vi "Get Sub-Item Type Descriptor.vi"(9 "error in (no error)":errorcluster, 10 ".NET AdsDataType":refnum<k24>) -> (1 "error out":errorcluster, 2 ".NET AdsDataType":refnum<k24>, 3 "[Sub-Item Type Descriptor]":T1[](array[typedef]))   [LabVIEW 2018, in "TwinCAT ADS.lvclass"]
uses:
  TwinCAT ADS.lvclass
  TwinCAT.Ads
  Controls/PLC Sub-Item Type Descriptor.ctl
  Controls/PLC Type.ctl
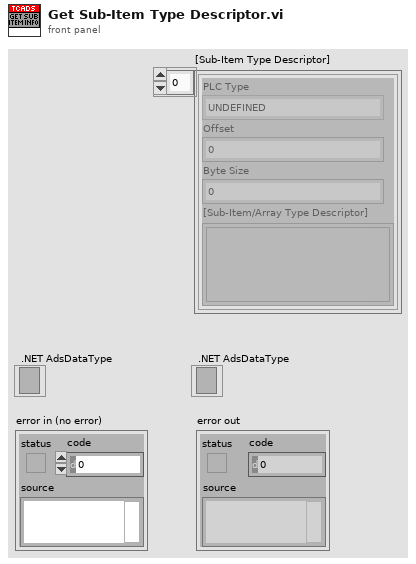
[diagram p1: front panel]
types:
  T1 = typedef "TwinCAT ADS.lvclass/PLC Sub-Item Type Descriptor.ctl" = cluster{"PLC Type":T2, "Offset":i32, "Byte Size":i32, "[Sub-Item/Array Type Descriptor]":variant[]}
  T2 = typedef "TwinCAT ADS.lvclass/PLC Type.ctl" = enum16{"UNDEFINED", "INT", "DINT", "REAL", "LREAL", "SINT", "BYTE", "UINT", "UDINT", "LINT", "ULINT", "STRING", "WSTRING", "BOOL", "TIME", "LTIME", "DATE", "DT", "TOD", "ARRAY", "JAGGED ARRAY", "STRUCT", "FUNCTION BLOCK", "POINTER", "USER DEFINED"}
  T3 = typedef "TwinCAT ADS.lvclass/PLC Array Type Descriptor.ctl" = cluster{"Fundamental PLC Type":T2, "Fundamental Type Byte Size":i32, "Item Count":i32, "Dimension Lengths":i32[], "Sub-Item Type Descriptor":variant}
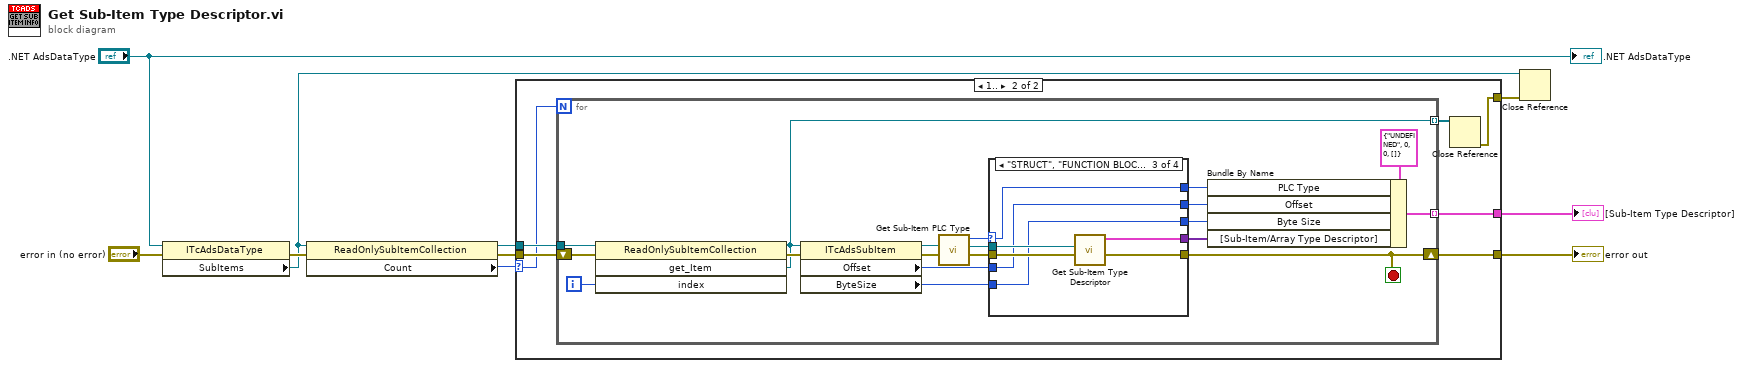
[diagram p0: block diagram]
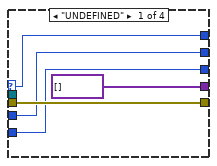
[diagram p3: hidden frame]
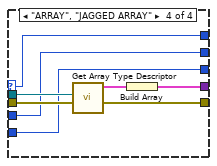
[diagram p5: hidden frame]
diagram:
  n1 = property class="ITcAdsDataType"(reference=".NET AdsDataType", error in="error in (no error)") -> (error out=w10:errorcluster, "SubItems"=w1:refnum<k24>)  [unwired: 1 out]
  n2 = property class="ReadOnlySubItemCollection"(reference=w1, error in=w10) -> (reference out=w7:refnum<k24>, error out=w8:errorcluster, "Count"=w4:i32)
  n3 = case shown="1.." w4 {
    selector: w4 -> [_ w14]
    tunnel: w8 -> [w11 w18]
    tunnel: w7 -> [_ w17]
    tunnel: [w11 w16] -> w6
    tunnel: [_ w15] -> w5
    tunnel: [_ w12] -> w2
    frame Default {
    }
    frame 1.. {
      n4 = for {
        N: w14 -> [_]
        shift-right: [w20] -> w16
        shift-left: w18 -> [w37]
        tunnel: w17 -> [w35]
        tunnel: [w26] -> w15 mode=indexing
        tunnel: [w21] -> w13 mode=indexing
        i -> [w36]
        stop <- w20 stop-if-true
        n5 = invoke class="ReadOnlySubItemCollection" method="get_Item"(reference=w35, error in=w37, "index"=w36) -> (error out=w34:errorcluster, "get_Item"=w21:refnum<k24>)  [unwired: 1 in, 2 out]
        n6 = property class="ITcAdsSubItem"(reference=w21, error in=w34) -> (reference out=w32:refnum<k24>, error out=w33:errorcluster, "Offset"=w19:i32, "ByteSize"=w28:i32)
        n7 = call "Get Sub-Item PLC Type.vi"("error in (no error)"=w33, ".NET AdsSubItem"=w32) -> ("error out"=w31:errorcluster, ".NET AdsSubItem"=w29:refnum<k24>, "PLC Type"=w30:T2)  [unwired: 7 in]
        n8 = case shown="\"STRUCT\", \"FUNCTION BLOCK\"" w30 {
          selector: w30 -> [w41 w45 w49 w58]
          tunnel: w31 -> [w42 w46 w53 w61]
          tunnel: w29 -> [_ _ w51 w59]
          tunnel: w19 -> [w40 w44 w48 w57]
          tunnel: w28 -> [w39 w43 w47 w56]
          tunnel: [w42 w46 w52 w60] -> w20
          tunnel: [variant[] [] ("[Sub-Item Type Information]") _ w50 w54] -> w25
          tunnel: [w39 w43 w47 w56] -> w24
          tunnel: [w40 w44 w48 w57] -> w23
          tunnel: [w41 w45 w49 w58] -> w22
          frame "UNDEFINED" {
          }
          frame Default {
          }
          frame "STRUCT", "FUNCTION BLOCK" {
            n9 = call "Get Sub-Item Type Descriptor.vi"("error in (no error)"=w53, ".NET AdsDataType"=w51) -> ("error out"=w52:errorcluster, "[Sub-Item Type Descriptor]"=w50:T1[])  [unwired: 7 in, 1 out]
          }
          frame "ARRAY", "JAGGED ARRAY" {
            n10 = call "Get Array Type Descriptor.vi"("error in (no error)"=w61, ".NET AdsDataType"=w59) -> ("error out"=w60:errorcluster, "Array Type Descriptor"=w55:T3)  [unwired: 7 in, 1 out]
            n11 = Build Array(w55) -> (w54:T3[])
          }
        }
        n12 = Bundle By Name(cluster=T1 {"PLC Type"=enum."UNDEFINED", "Offset"=0, "Byte Size"=0, "[Sub-Item/Array Type Descriptor]"=[]} ("Sub-Item Type Information"), "PLC Type"=w22, "Offset"=w23, "Byte Size"=w24, "[Sub-Item/Array Type Descriptor]"=w25) -> (w26:T1)
      }
      n13 = Close Reference(reference=w13) -> (error out=w12:errorcluster)  [unwired: 1 in]
    }
  }
  "error out" <- w6
  "[Sub-Item Type Descriptor]" <- w5
  n14 = Close Reference(reference=w1, error in (no error)=w2) -> ()  [unwired: 1 out]
  ".NET AdsDataType" <- ".NET AdsDataType"
